vi "Configure Offset Level.vi"(7 "Mode":T2 items=["AC", "DC"], 8 "error in (no error)":errorcluster, 9 "Offset Level [A]":dbl min=0.0 max=0.03 step=0.001 format="%_4p", 10 "Step":T1=1 min=1 max=99 step=1, 11 "VISA resource name":refnum<visa-resource-name>) -> (0 "error out":errorcluster, 3 "VISA resource name out":refnum<visa-resource-name>)   [LabVIEW 2025, in "Chroma 19052.lvlib"]
uses:
  <instrlib>/Chroma 19052/Public/Utility/Type Def/AC-DC modes--ring.ctl
  <instrlib>/Chroma 19052/Public/Utility/Type Def/steps--numeric.ctl
  <instrlib>/Chroma 19052/Chroma 19052.lvlib
panel:
  # "Configure Offset Level"
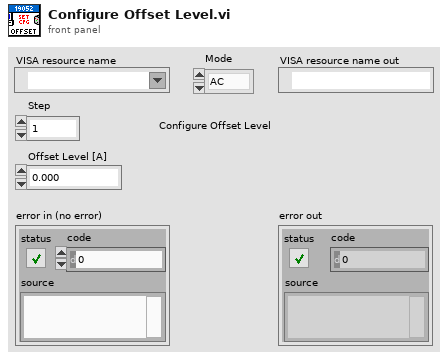
[diagram p1: front panel]
types:
  T1 = typedef "Chroma 19052.lvlib/steps--numeric.ctl" = u8
  T2 = typedef "AC-DC modes--ring.ctl" = i32
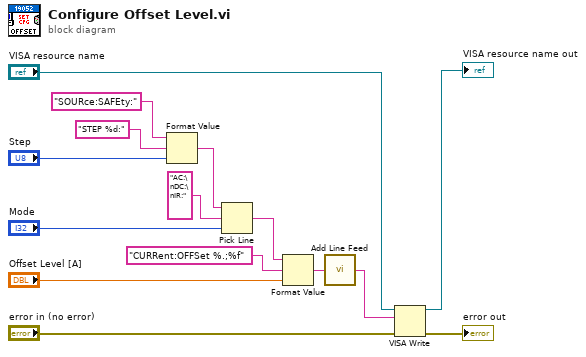
[diagram p0: block diagram]
diagram:
  n1 = Format Value(string ("")="SOURce:SAFEty:", format string="STEP %d:", value (0)="Step") -> (output string=w8:string)
  n2 = Pick Line(string ("")=w8, multi-line string="AC:\nDC:\nIR:", line index="Mode") -> (output string=w7:string)
  n3 = Format Value(string ("")=w7, format string="CURRent:OFFSet %.;%f", value (0)="Offset Level [A]") -> (output string=w6:string)
  n4 = call <instrlib>:"Add Line Feed.vi"("Command string"=w6) -> ("Concatenated string"=w5:string)  [unwired: 4 in]
  n5 = VISA Write(VISA resource name="VISA resource name", write buffer=w5, error in (no error)="error in (no error)") -> (VISA resource name out=→"VISA resource name out":refnum<visa-resource-name>, error out=→"error out":errorcluster)  [unwired: 1 out]
